vi "Empty Task Map.vi"() -> (0 "Task Map":map{string, refnum<k21>}(c390))   [LabVIEW 2021, in "Load Frame.lvlib"]
doc: "Create an empty DAQmx Task Map where keys are strings and values are Tasks."
uses:
  Load Frame.lvlib
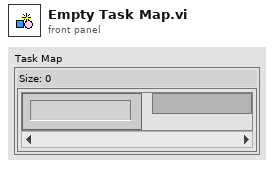
[diagram p1: front panel]
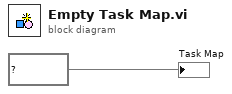
[diagram p0: block diagram]
diagram:
  "Task Map" <- map{string, refnum<k21>} {} ("Size: 0")
